vi "PH_Sequencer.evt call PP Timeout SM.vi"(0 "i ref in":refnum<vi>, 2 "Instance":string="N/A", 3 "Power Unit":T2, 4 "PP Timeout SM":T1, 5 "error in (no error)":errorcluster) -> (14 "i ref out":refnum<vi>, 19 "error out":errorcluster)   [LabVIEW 2014, in "PH_Sequencer.lvlib"]
doc: "This VI calls for PPTimeoutSM by a simple call."
uses:
  PH_Sequencer.lvlib
  PH_PP_Common/PH_PP_Common.PUs.ctl
  PH_PowerUnit_BaseClass/PH_PowerUnit_BaseClass.SM States.ctl
  CSCore/CSSystem/CoreLib/CoreLib.short 2 byte array.vi
  CSCore/CSSystem/CoreLib/CoreLib.lvlib
  CSCore/BaseProcess/BaseProcess.lvlib
  PH_PP_Common/PH_PP_Common.lvlib
  PH_PowerUnit_BaseClass/PH_PowerUnit_BaseClass.lvlib
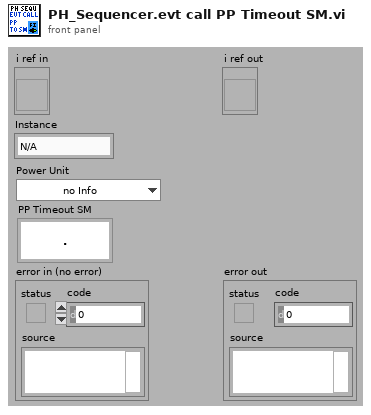
[diagram p1: front panel]
types:
  T1 = typedef "PH_PowerUnit_BaseClass.lvlib/PH_PowerUnit_BaseClass.SM States.ctl" = enum16{".", "Stand by", "Switch PU on", "Configure", "Set Default Voltage", "Set STANDBY", "Set READY", "Wait for Shot Cmd", "Open Dump Rods", "Open Ross Relais", "Close Ross Relais", "Switch PSU on", "Switch PSU off", "Charge", "Switch GD Channel on", "Close Dump Rods", "Rods-TO", "RR-TO", "PSU-TO", "Trigger-TO"}
  T2 = typedef "PH_PP_Common.lvlib/PH_PP_Common.PUs.ctl" = enum16{"no Info", "PA-19mm-1", "PA-19mm-2", "PA-45mm-PILC", "PA-45mm-MAIN", "MA-PU-1", "MA-PU-2", "MA-PU-3", "MA-PU-4", "MA-PU-5", "MA-PU-6", "MA-FR", "MA-PILC", "PA-45mm-DP"}
  T3 = typedef "CoreDefs.rawDataType.ctl" = i8[]
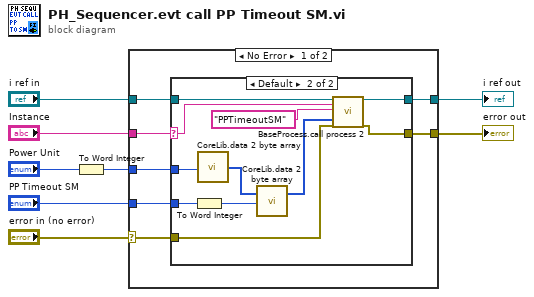
[diagram p0: block diagram]
diagram:
  n1 = To Word Integer(number="Power Unit") -> (16bit integer=w1:i16)
  n2 = case shown="No Error" "error in (no error)" {
    selector: "error in (no error)" -> [w12 w29]
    tunnel: [w15 w30] -> w3
    tunnel: [w14 w29] -> w2
    tunnel: "i ref in" -> [w13 w30]
    tunnel: "Instance" -> [w11 _]
    tunnel: w1 -> [w10 _]
    tunnel: "PP Timeout SM" -> [w9 _]
    frame No Error {
      n3 = case shown="Default" w11 {
        selector: w11 -> [_ w19]
        tunnel: [w17 w27] -> w15
        tunnel: [w16 w26] -> w14
        tunnel: w13 -> [w17 w25]
        tunnel: w12 -> [w16 w24]
        tunnel: w10 -> [_ w21]
        tunnel: w9 -> [_ w20]
        frame "N/A" {
        }
        frame Default {
          n4 = To Word Integer(number=w20) -> (16bit integer=w18:i16)
          n5 = call-poly "CoreLib.data 2 byte array.vi"("i16"=w21) -> ("byteArray out"=w23:T3)  [unwired: 18 in]
          n6 = call-poly "CoreLib.data 2 byte array.vi"("byteArray"=w23, "i16"=w18) -> ("byteArray out"=w22:T3)  [unwired: 17 in]
          n7 = call "BaseProcess.call process 2.vi"("i ref in"=w25, "Object"=w19, "Selector"="PPTimeoutSM", "Data"=w22, "error in (no error)"=w24) -> ("i ref out"=w27:refnum<vi>, "error out"=w26:errorcluster)  [unwired: 13 in]
        }
      }
    }
    frame Error {
    }
  }
  "error out" <- w2
  "i ref out" <- w3
